vi "Switch.vi"() -> ()   [LabVIEW 2016]
panel:
  out "Boolean":bool
  in  "stop":bool
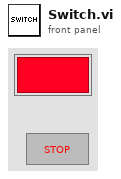
[diagram p1: front panel]
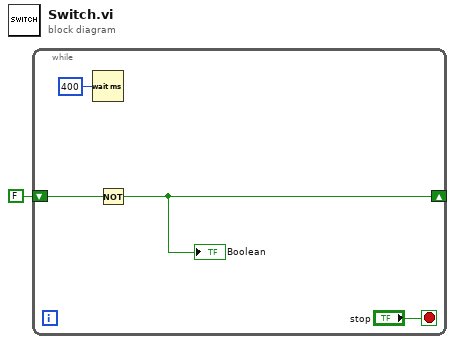
[diagram p0: block diagram]
diagram:
  n1 = while {
    shift-right: [w2] -> _
    shift-left: FALSE ("Start") -> [w3]
    stop <- "stop" stop-if-true
    n2 = Wait (ms)(milliseconds to wait=u32 400) -> ()  [unwired: 1 out]
    n3 = Not(x=w3) -> (.not. x?=w2:bool)
    "Boolean" <- w2
  }
